vi "GlobalVariables.vi"() -> ()   [LabVIEW 2016]
uses:
  <vilib>/vision/Image Controls.llb/IMAQ Image.ctl
panel:
  out "Toup Ref Img":T1
  out "Toup Temp Img":T1
  out "Toup Resolution":cluster{"pWidth":i32, "pHeight":i32}
  out "Toup Event":refnum<event-registration>
  in  "Toup Handle":i32
  in  "Orca Buffer":T2
  in  "Orca Valid":bool
  in  "Orca Handle":u32
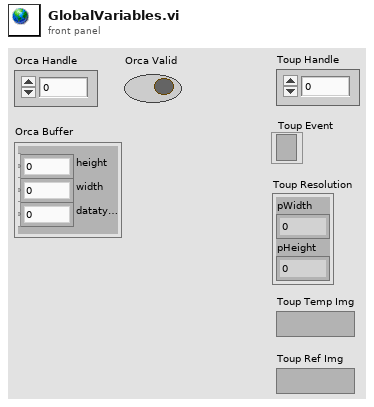
[diagram p1: front panel]
types:
  T1 = typedef "IMAQ Image.ctl" = refnum<image>
  T2 = cluster{"height":u32, "width":u32, "datatype":u32}
diagram:
